vi "Enumerate DVR Items.vi"(11 "Class":T4 caption="Object") -> (2 "Type Tree":T1[](array[typedef]), 3 "LVClassLibrary":refnum<vi>)   [LabVIEW 2018, in "LVClassByRef.lvlib"]
uses:
  <resource>/Framework/Providers/LVClassByRef/LVClassByRef.lvlib
  <resource>/Framework/Providers/API/ItemRef.ctl
  <resource>/Framework/Providers/LVClassByRef/Type Item.ctl
  <resource>/Framework/Providers/LVClassByRef/Tree Item.ctl
  <vilib>/Utility/Data Type/Type Definitions/Data Type.ctl
  <vilib>/Utility/Data Type/NI_Data Type.lvlib
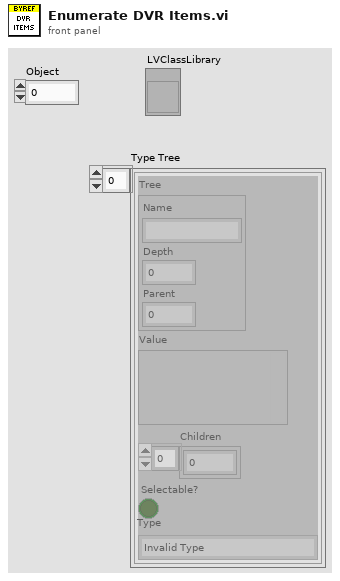
[diagram p1: front panel]
types:
  T1 = typedef "LVClassByRef.lvlib/Type Item.ctl" = cluster{"Tree":T2, "Value":variant, "Children":i32[], "Selectable?":bool, "Type":T3}
  T2 = typedef "LVClassByRef.lvlib/Tree Item.ctl" = cluster{"Name":string, "Depth":i32, "Parent":i32}
  T3 = typedef "NI_Data Type.lvlib/Data Type.ctl" = enum8{"Invalid Type", "Void", "I8", "I16", "I32", "I64", "U8", "U16", "U32", "U64", "Single Float", "Double Float", "Extended Float", "Single Complex", "Double Complex", "Extended Complex", "Enum U8", "Enum U16", "Enum U32", "Enum U64", "Single Float With Unit", "Double Float With Unit", "Extended Float With Unit", "Single Complex with Unit", "Double Complex with Unit", "Extended Complex with Unit", "Boolean", "String", "Path", "Picture", "Tag", "Array", "Cluster", "Variant", "LV Variant", "Waveform", "Timestamp", "Digital Waveform", "Digital Data", "ExpressData", "Refnum", "External Data", "VI", "Poly VI", "LabVIEW Class Instance", "Fixed Point"}
  T4 = typedef "ItemRef.ctl" = u64
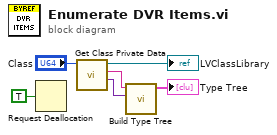
[diagram p0: block diagram]
diagram:
  n1 = Request Deallocation(TRUE ("flag")) -> ()
  n2 = call <resource>:"Get Class Private Data.vi"("Class"="Class") -> ("Value"=w3:variant, "Name"=w4:string, "LVClassLibrary"=→"LVClassLibrary":refnum<vi>)  [unwired: 8 in]
  n3 = call <resource>:"Build Type Tree.vi"("Value"=w3, "Name"=w4) -> ("Type Tree"=→"Type Tree":T1[])  [unwired: 9 in]
